vi "Destroy Current Value Table.vi"(8 "error in (no error)":errorcluster, 11 "Current Value Table":T1) -> (0 "error out":errorcluster)   [LabVIEW 2015, in "CurrentValueTable.lvlib" / "CurrentValueTable.lvclass"]
uses:
  CurrentValueTable.lvclass
  CurrentValueTable Reference.ctl
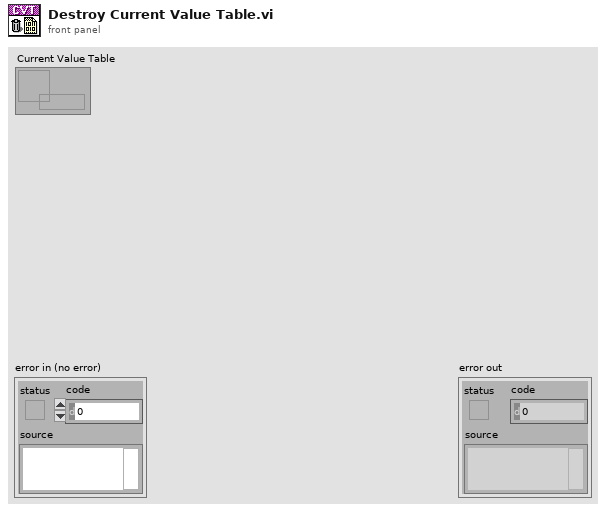
[diagram p1: front panel]
types:
  T1 = typedef "CurrentValueTable.lvlib/CurrentValueTable.lvclass/CurrentValueTable Reference.ctl" = refnum<data-value>
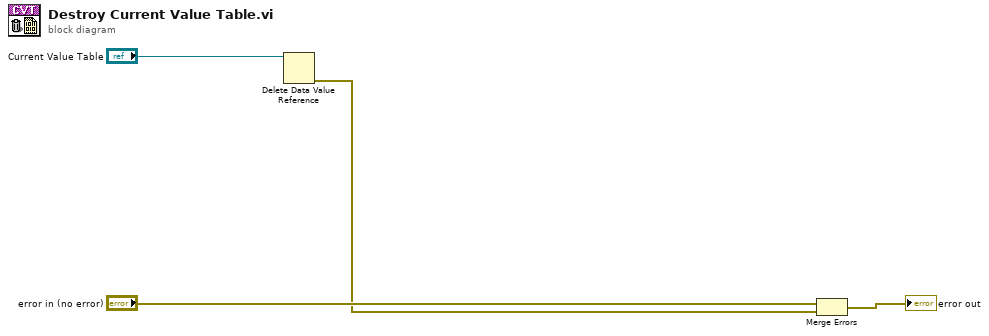
[diagram p0: block diagram]
diagram:
  n1 = Delete Data Value Reference(data value reference="Current Value Table") -> (error out=w1:errorcluster)  [unwired: 1 in, 1 out]
  n2 = Merge Errors("error in (no error)", w1) -> (→"error out":errorcluster)
